vi "To Test Event.vi"(11 "TestManagerMsg.Test in":refnum<class "TestManagerMsg.Test.lvclass">) -> (3 "Test Registration":T1)   [LabVIEW 2013, in "Caraya.lvlib" / "TestManagerMsg.Test.lvclass"]
uses:
  TestManagerMsg.Test.lvclass
  Test Result/Test Registration Data.ctl
  Test Manager Message/TestManagerMsg.lvclass/TestManagerMsg.ctl
  Test Manager Message/TestManagerMsg.lvclass
  Test Result/Test Result.lvclass
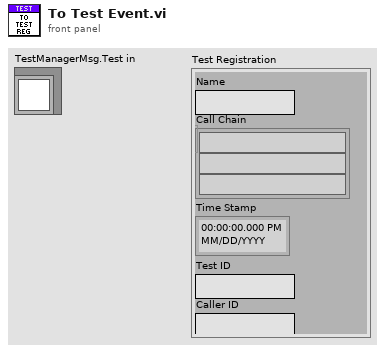
[diagram p1: front panel]
types:
  T1 = typedef "Caraya.lvlib/Test Result.lvclass/Test Registration Data.ctl" = cluster{"Name":string, "Call Chain":string[], "Time Stamp":timestamp, "Test ID":string, "Caller ID":string}
  T2 = typedef "Caraya.lvlib/TestManagerMsg.Test.lvclass/Test-Data -- cluster.ctl" = cluster{"test-name":string, "call-chain":string[], "timestamp":timestamp}
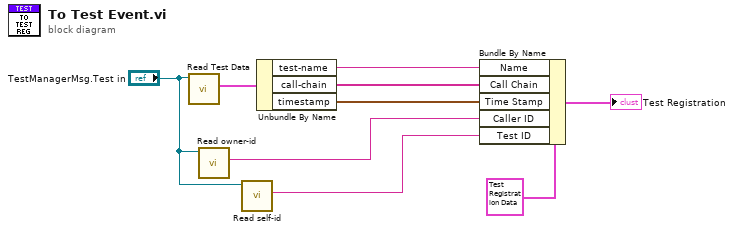
[diagram p0: block diagram]
diagram:
  n1 = call "Read Test Data.vi"("Message Test"="TestManagerMsg.Test in") -> ("Test Data"=w5:T2)  [unwired: 9 in, 1 out]
  n2 = call "Read owner-id.vi"("TestManagerMsg in"="TestManagerMsg.Test in") -> ("owner-id"=w9:string)  [unwired: 9 in, 1 out]
  n3 = call "Read self-id.vi"("TestManagerMsg in"="TestManagerMsg.Test in") -> ("self-id"=w1:string)  [unwired: 9 in, 1 out]
  n4 = Unbundle By Name(w5) -> ("test-name"=w6:string, "call-chain"=w8:string[], "timestamp"=w7:timestamp)
  n5 = Bundle By Name(cluster=T1 {"Name"="", "Call Chain"=[], "Time Stamp"=timestamp(0 s since 1904-01-01), "Test ID"="", "Caller ID"=""} ("Test Registration"), "Name"=w6, "Call Chain"=w8, "Time Stamp"=w7, "Caller ID"=w9, "Test ID"=w1) -> (→"Test Registration":T1)
